vi "robot set drag teach.vi"(8 "error in (no error)":errorcluster caption="错误输入（无错误）", 10 "enable":bool, 11 "robot_id":i32) -> (0 "error out":errorcluster caption="错误输出", 2 "function return":i32, 3 "robot_id out":i32, 4 "x != 0?":bool)   [LabVIEW 2020]
uses:
  small_scara_interface.dll
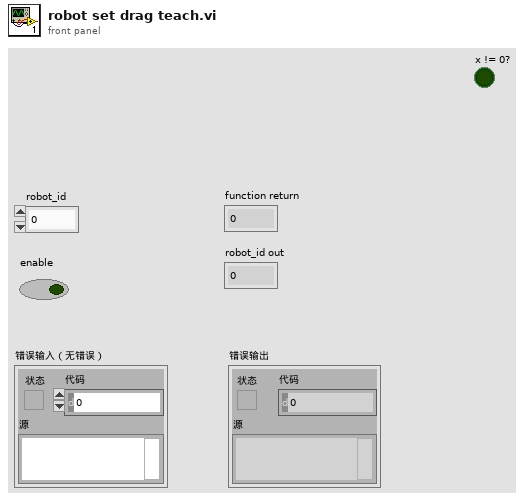
[diagram p1: front panel]
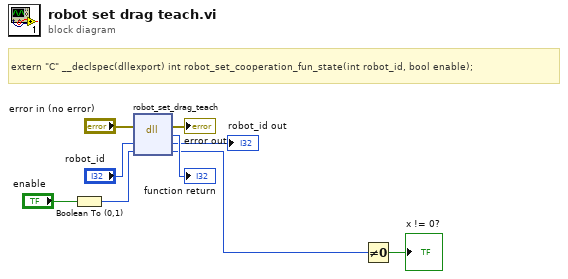
[diagram p0: block diagram]
diagram:
  # "extern \"C\" __declspec(dllexport) int robot_set_cooperation_fun_state(int robot_id, bool enable);"
  n1 = Boolean To (0,1)(Boolean="enable") -> (0, 1=w6:i16)
  n2 = dll-call lib="C:/Users/Mogroup-3/Desktop/labview multichannel v314/subvi/robot/subvi/Robot-HL/small_scara_interface/small_scara_interface.dll" fn="robot_set_drag_teach"(error in="error in (no error)", "robot_id"="robot_id", "enable"=w6) -> (error out=→"error out":errorcluster, "返回类型"=→"function return":i32, "robot_id"=→"robot_id out":i32, "enable"=w2:u8)  [unwired: 2 in, 1 out]
  n3 = Not Equal To 0?(x=w2) -> (x != 0?=→"x != 0?":bool)
